vi "Get FPGA Ref.vi"(8 "error in":errorcluster, 11 "nPAS in":refnum<class "nPAS.lvclass">) -> (0 "error out":errorcluster, 2 "FPGA Ref":T1, 3 "nPAS out":refnum<class "nPAS.lvclass">)   [LabVIEW 2017, in "gPAS Library.lvlib" / "nPAS.lvclass"]
uses:
  nPAS.lvclass
  FPGA Ref.ctl
  Session/Raw FPGA/FPGA Session.lvclass
  nPAS.lvclass/nPAS.ctl
  Session/Raw FPGA/FPGA Session.lvclass/FPGA Session.ctl
  Session/Raw FPGA/Read FPGA Ref.vi
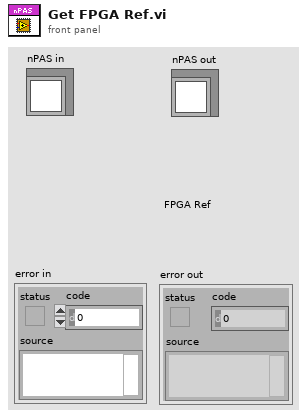
[diagram p1: front panel]
types:
  T1 = typedef "FPGA Ref.ctl" = refnum<k20>
  T2 = typedef "Session - Root.lvclass/Session Handle.ctl" = refnum<data-value>
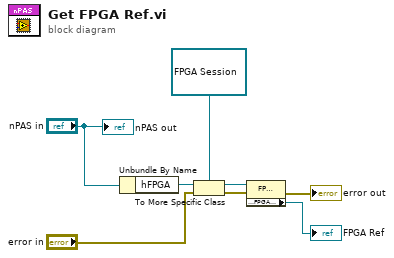
[diagram p0: block diagram]
diagram:
  n1 = Unbundle By Name("nPAS in") -> ("hFPGA"=w6:T2)
  n2 = To More Specific Class(target class=refnum<data-value> refnum ("hFPGA"), reference=w6, error in="error in") -> (specific class reference=w4:refnum<data-value>, error out=w8:errorcluster)
  n3 = property class="FPGA Session"(reference=w4, error in=w8) -> (error out=→"error out":errorcluster, "Accessors:FPGA Ref"=→"FPGA Ref":T1)  [unwired: 1 out]
  "nPAS out" <- "nPAS in"
